vi "ScalingLockLogic.vi"   [LabVIEW 2016]
uses:
  <vilib>/Rock Robotics/WPI/Solenoid/WPI_SolenoidValue.ctl
  <vilib>/Rock Robotics/WPI/Solenoid/WPI_SolenoidSetEnum.vi
  Robot Global Data.vi
  <vilib>/Rock Robotics/WPI/Solenoid/Deprecated/WPI_SolenoidGetBool.vi
  <vilib>/Rock Robotics/WPI/Solenoid/Deprecated/WPI_SolenoidSetBool.vi
  <vilib>/Rock Robotics/Network Tables/NT Write Boolean.vi
types:
  T1 = typedef "WPI_SolenoidValue.ctl" = enum16{"Off", "On", "Forward", "Reverse"}
  T2 = typedef "WPI_SolenoidDevRef.ctl" = cluster{"DevStatus":errorcluster, "Pneumatics Control Module":u8, "Forward Solenoid Channel":T3, "Reverse Solenoid Channel":T3}
  T3 = typedef "WPI_SolenoidChannel.ctl" = enum8{"Solenoid 0", "Solenoid 1", "Solenoid 2", "Solenoid 3", "Solenoid 4", "Solenoid 5", "Solenoid 6", "Solenoid 7", "Invalid"}
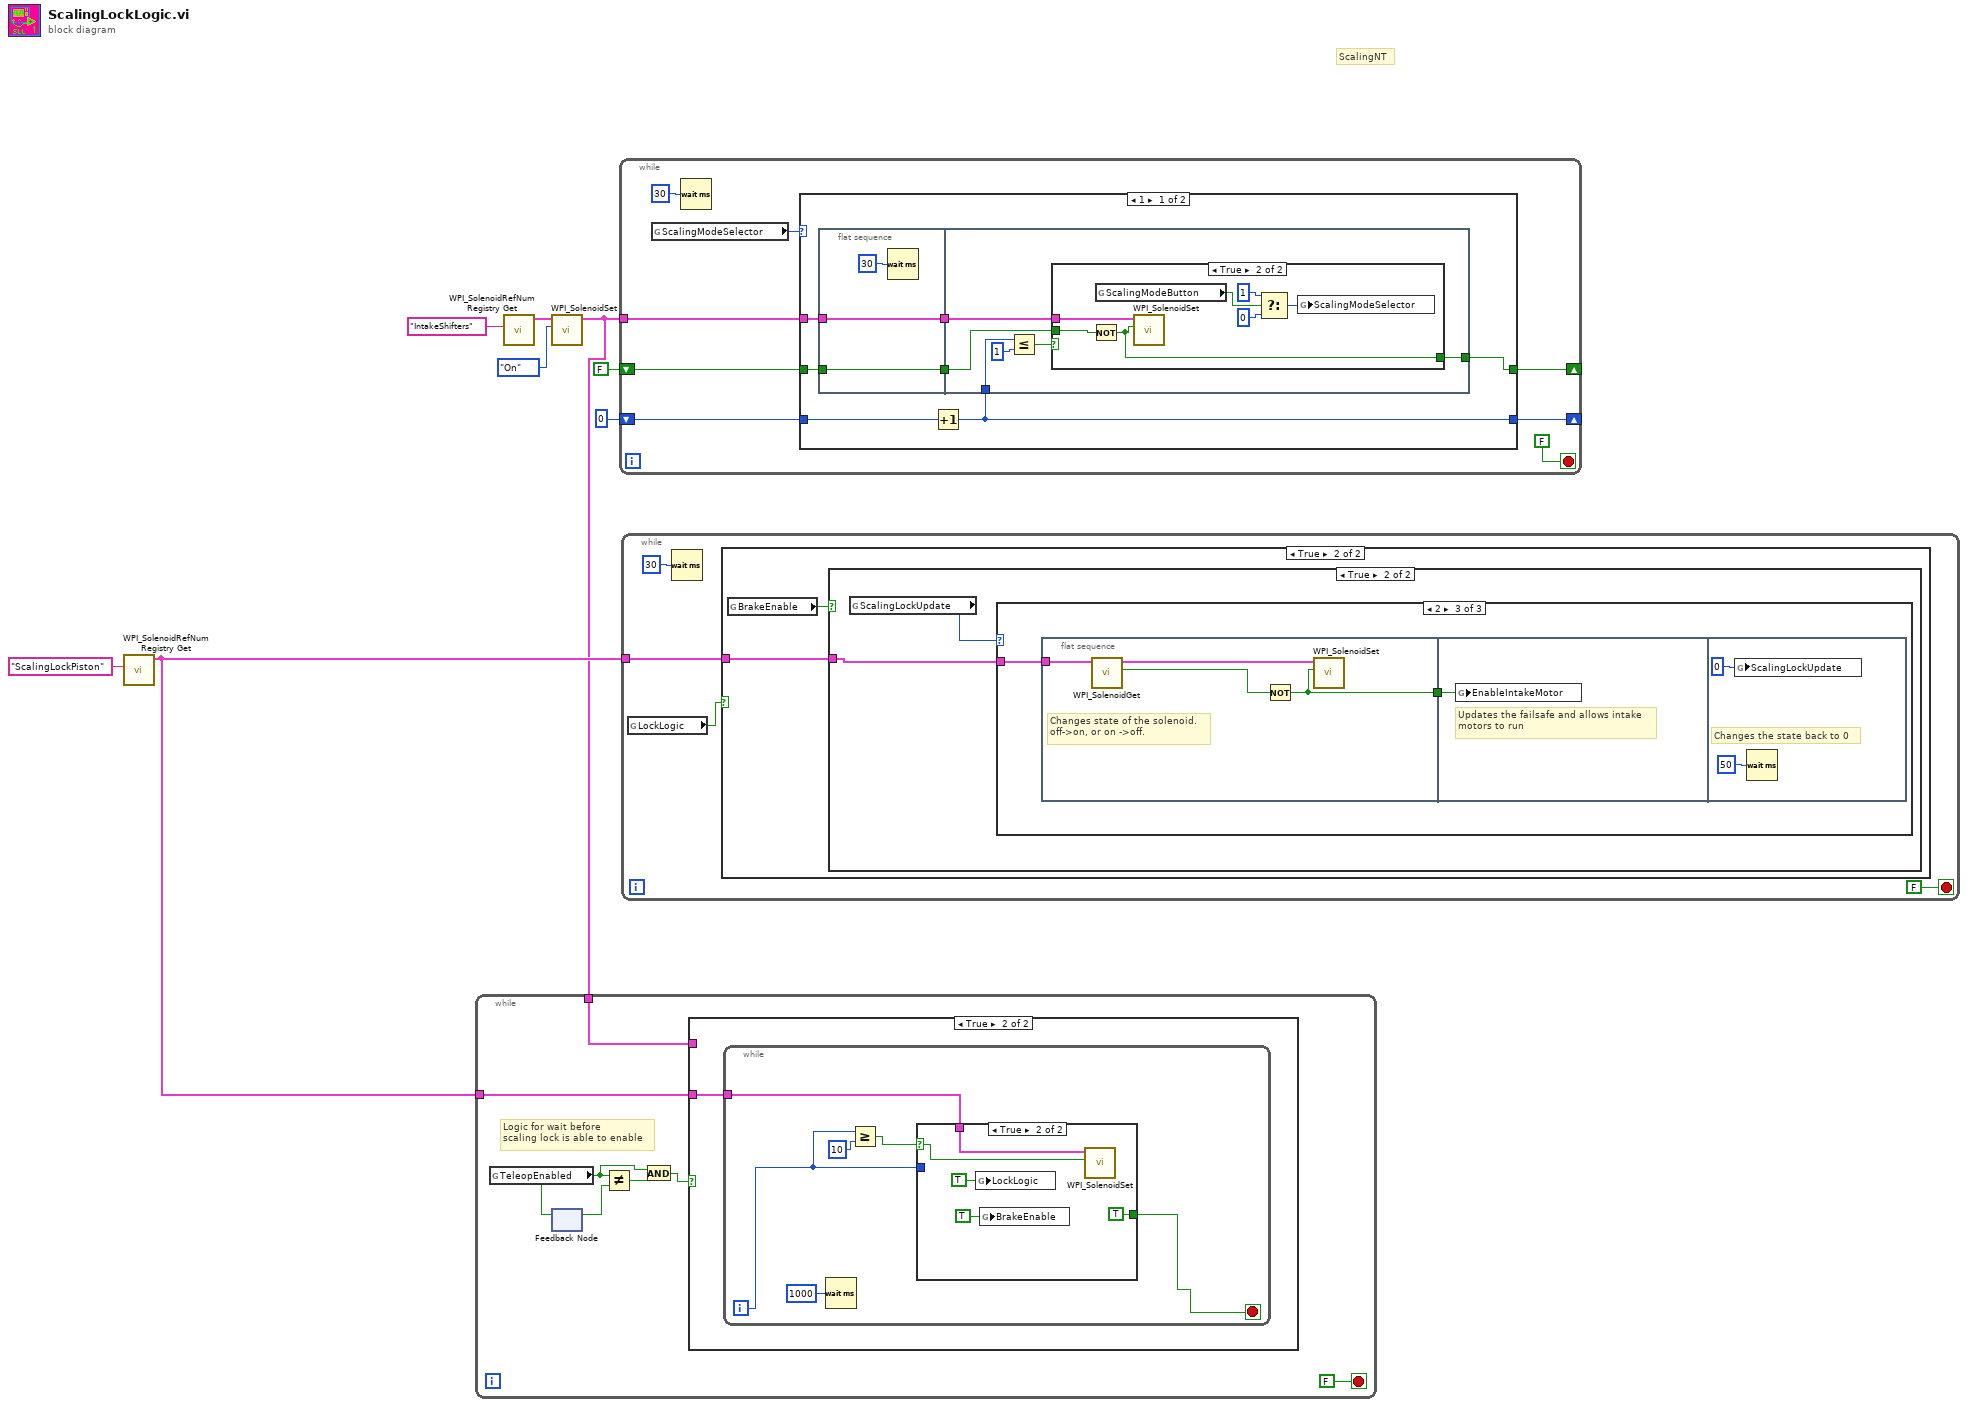
[diagram p0: block diagram]
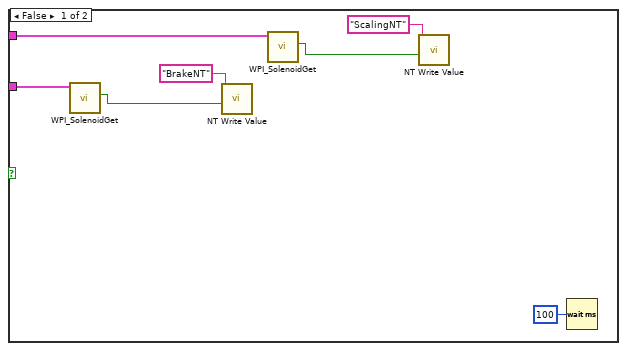
[diagram p2: hidden frame]
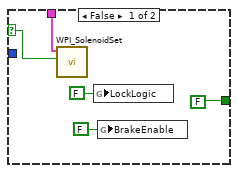
[diagram p3: hidden frame]
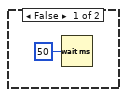
[diagram p4: hidden frame]
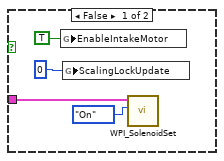
[diagram p5: hidden frame]
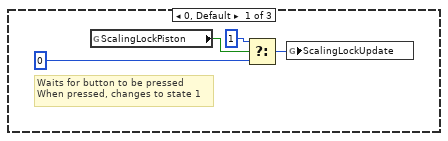
[diagram p6: hidden frame]
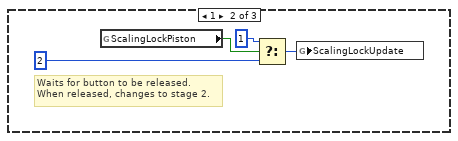
[diagram p7: hidden frame]
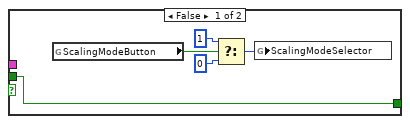
[diagram p8: hidden frame]
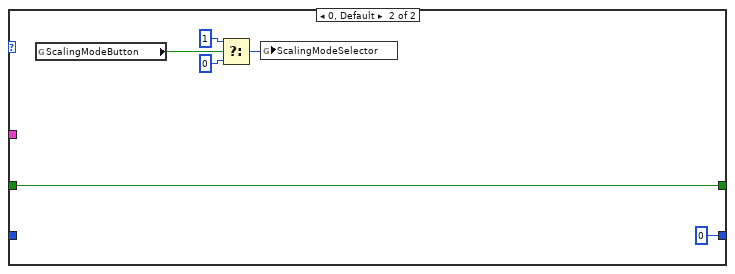
[diagram p9: hidden frame]
diagram:
  # "ScalingNT"
  n1 = call <vilib>:"WPI_SolenoidRefNum Registry Get.vi"("refnum name"="ScalingLockPiston") -> ("SolenoidDevRef"=w3:T2)  [unwired: 9 in, 1 out]
  n2 = call <vilib>:"WPI_SolenoidRefNum Registry Get.vi"("refnum name"="IntakeShifters") -> ("SolenoidDevRef"=w5:T2)  [unwired: 9 in, 1 out]
  n3 = call-poly <vilib>:"WPI_SolenoidSet.vi"("Value"=WPI_SolenoidValue."On", "SolenoidDevRef"=w5) -> ("SolenoidDevRef"=w1:T2)  [unwired: 8 in, 1 out]
  n4 = while {
    tunnel: w3 -> [w15]
    tunnel: w1 -> [w9]
    stop <- FALSE stop-if-true
    # "Logic for wait before \nscaling lock is able to enable"
    n5 = global read "Robot Global Data.vi" "TeleopEnabled"() -> (w11:bool)
    n6 = feedback-in #1(w11) -> ()
    n7 = feedback #1() -> (w13:bool)  [unwired: 1 in]
    n8 = Not Equal?(x=w11, y=w13) -> (x != y?=w12:bool)
    n9 = And(x=w11, y=w12) -> (x .and. y?=w10:bool)
    n10 = case shown="True" w10 {
      tunnel: w15 -> [w16 w23]
      tunnel: w9 -> [w18 _]
      frame False {
        n11 = call-poly <vilib>:"WPI_SolenoidGet.vi"("SolenoidDevRef"=w16) -> ("Value"=w17:bool)  [unwired: 8 in, 2 out]
        n12 = call-poly <vilib>:"NT Write Value.vi"("Boolean"=w17, "Name"="BrakeNT") -> ()  [unwired: 9 in, 1 out]
        n13 = call-poly <vilib>:"WPI_SolenoidGet.vi"("SolenoidDevRef"=w18) -> ("Value"=w19:bool)  [unwired: 8 in, 2 out]
        n14 = call-poly <vilib>:"NT Write Value.vi"("Boolean"=w19, "Name"="ScalingNT") -> ()  [unwired: 9 in, 1 out]
        n15 = Wait (ms)(milliseconds to wait=u32 100) -> ()  [unwired: 1 out]
      }
      frame True {
        n16 = while {
          tunnel: w23 -> [w25]
          i -> [w27]
          stop <- w24 stop-if-true
          n17 = Wait (ms)(milliseconds to wait=u32 1000) -> ()  [unwired: 1 out]
          n18 = Greater Or Equal?(x=w27, y=10) -> (x >= y?=w28:bool)
          n19 = case shown="True" w28 {
            selector: w28 -> [w31 w39]
            tunnel: w27 -> [_ _]
            tunnel: w25 -> [w30 w37]
            tunnel: [FALSE TRUE] -> w24
            frame False {
              n20 = call-poly <vilib>:"WPI_SolenoidSet.vi"("Value"=w31, "SolenoidDevRef"=w30) -> ()  [unwired: 8 in, 2 out]
              n21 = global write "Robot Global Data.vi" "LockLogic"(FALSE ("LockLogic")) -> ()
              n22 = global write "Robot Global Data.vi" "BrakeEnable"(FALSE ("BrakeEnable")) -> ()
            }
            frame True {
              n23 = global write "Robot Global Data.vi" "LockLogic"(TRUE ("LockLogic")) -> ()
              n24 = global write "Robot Global Data.vi" "BrakeEnable"(TRUE ("BrakeEnable")) -> ()
              n25 = call-poly <vilib>:"WPI_SolenoidSet.vi"("Value"=w39, "SolenoidDevRef"=w37) -> ()  [unwired: 8 in, 2 out]
            }
          }
        }
      }
    }
  }
  n26 = while {
    shift-right: [w45] -> _
    shift-left: FALSE -> [w43]
    tunnel: w1 -> [w42]
    shift-right: [w41] -> _
    shift-left: 0 -> [w40]
    stop <- FALSE stop-if-true
    n27 = global read "Robot Global Data.vi" "ScalingModeSelector"() -> (w46:i32)
    n28 = Wait (ms)(milliseconds to wait=u32 30) -> ()  [unwired: 1 out]
    n29 = case shown="1" w46 {
      tunnel: [w48 w77] -> w45
      tunnel: w43 -> [w53 w77]
      tunnel: w42 -> [w52 _]
      tunnel: [w50 0] -> w41
      tunnel: w40 -> [w51 _]
      frame 1 {
        n30 = flat-sequence {
          tunnel: [w56] -> w54
          tunnel: w53 -> [w56]
          tunnel: w52 -> [w55]
          tunnel: [w55] -> w49
          tunnel: w54 -> [w59]
          tunnel: w50 -> [w61]
          tunnel: w49 -> [w60]
          tunnel: [w58] -> w48
          frame #0 {
            n31 = Wait (ms)(milliseconds to wait=u32 30) -> ()  [unwired: 1 out]
          }
          frame #1 {
            n32 = Less Or Equal?(x=w61, y=1) -> (x <= y?=w63:bool)
            n33 = case shown="True" w63 {
              tunnel: w59 -> [w64 w75]
              tunnel: w60 -> [_ w70]
              tunnel: [w64 w69] -> w58
              frame False {
                n34 = global read "Robot Global Data.vi" "ScalingModeButton"() -> (w65:bool)
                n35 = Select(t=1, s=w65, f=0) -> (s? t:f=w67:i32)
                n36 = global write "Robot Global Data.vi" "ScalingModeSelector"(w67) -> ()
              }
              frame True {
                n37 = Not(x=w75) -> (.not. x?=w69:bool)
                n38 = global read "Robot Global Data.vi" "ScalingModeButton"() -> (w74:bool)
                n39 = call-poly <vilib>:"WPI_SolenoidSet.vi"("Value"=w69, "SolenoidDevRef"=w70) -> ()  [unwired: 8 in, 2 out]
                n40 = Select(t=1, s=w74, f=0) -> (s? t:f=w72:i32)
                n41 = global write "Robot Global Data.vi" "ScalingModeSelector"(w72) -> ()
              }
            }
          }
        }
        n42 = Increment(x=w51) -> (x+1=w50:i32)
      }
      frame 0, Default {
        n43 = global read "Robot Global Data.vi" "ScalingModeButton"() -> (w81:bool)
        n44 = Select(t=1, s=w81, f=0) -> (s? t:f=w79:i32)
        n45 = global write "Robot Global Data.vi" "ScalingModeSelector"(w79) -> ()
      }
    }
  }
  n46 = while {
    tunnel: w3 -> [w84]
    stop <- FALSE stop-if-true
    n47 = global read "Robot Global Data.vi" "LockLogic"() -> (w82:bool)
    n48 = Wait (ms)(milliseconds to wait=u32 30) -> ()  [unwired: 1 out]
    n49 = case shown="True" w82 {
      tunnel: w84 -> [_ w87]
      frame False {
        n50 = Wait (ms)(milliseconds to wait=u32 50) -> ()  [unwired: 1 out]
      }
      frame True {
        n51 = global read "Robot Global Data.vi" "BrakeEnable"() -> (w88:bool)
        n52 = case shown="True" w88 {
          tunnel: w87 -> [w89 w93]
          frame False {
            n53 = global write "Robot Global Data.vi" "EnableIntakeMotor"(TRUE ("EnableIntakeMotor")) -> ()
            n54 = global write "Robot Global Data.vi" "ScalingLockUpdate"(0) -> ()
            n55 = call-poly <vilib>:"WPI_SolenoidSet.vi"("Value"=WPI_SolenoidValue."On", "SolenoidDevRef"=w89) -> ()  [unwired: 8 in, 2 out]
          }
          frame True {
            n56 = global read "Robot Global Data.vi" "ScalingLockUpdate"() -> (w94:i32)
            n57 = case shown="2" w94 {
              tunnel: w93 -> [_ _ w103]
              frame 0, Default {
                # "Waits for button to be pressed\nWhen pressed, changes to state 1"
                n58 = global read "Robot Global Data.vi" "ScalingLockPiston"() -> (w98:bool)
                n59 = Select(t=1, s=w98, f=0) -> (s? t:f=w95:i32)
                n60 = global write "Robot Global Data.vi" "ScalingLockUpdate"(w95) -> ()
              }
              frame 1 {
                # "Waits for button to be released.\nWhen released, changes to stage 2."
                n61 = global read "Robot Global Data.vi" "ScalingLockPiston"() -> (w102:bool)
                n62 = Select(t=1, s=w102, f=2) -> (s? t:f=w99:i32)
                n63 = global write "Robot Global Data.vi" "ScalingLockUpdate"(w99) -> ()
              }
              frame 2 {
                n64 = flat-sequence {
                  tunnel: [w105] -> w104
                  tunnel: w103 -> [w107]
                  tunnel: w104 -> [w109]
                  frame #0 {
                    # "Changes state of the solenoid.\noff->on, or on ->off."
                    n65 = call-poly <vilib>:"WPI_SolenoidGet.vi"("SolenoidDevRef"=w107) -> ("Value"=w106:bool, "SolenoidDevRef"=w108:T2)  [unwired: 8 in, 1 out]
                    n66 = Not(x=w106) -> (.not. x?=w105:bool)
                    n67 = call-poly <vilib>:"WPI_SolenoidSet.vi"("Value"=w105, "SolenoidDevRef"=w108) -> ()  [unwired: 8 in, 2 out]
                  }
                  frame #1 {
                    # "Updates the failsafe and allows intake\nmotors to run"
                    n68 = global write "Robot Global Data.vi" "EnableIntakeMotor"(w109) -> ()
                  }
                  frame #2 {
                    # "Changes the state back to 0"
                    n69 = global write "Robot Global Data.vi" "ScalingLockUpdate"(0) -> ()
                    n70 = Wait (ms)(milliseconds to wait=u32 50) -> ()  [unwired: 1 out]
                  }
                }
              }
            }
          }
        }
      }
    }
  }
